vi "Save String Data to file.vi"(0 "Path":path, 5 "String to save":string, 7 "Header":string, 9 "Additional String":string, 12 "Disconnecting":bool) -> ()   [LabVIEW 2011]
panel:
  # "This vi saves data to file in a standard format\nData comes in as a 1D string\nA header is optional\nAn additional string can be added at the end of each line.\nThe path is the location of the data file.\n\n\nThe file is kept open at all times. When the software is to stop,\nthe disconnect is used to close the file properly.\nEvery 30 seconds, the file is flushed to empty the file buffer and\nforce the data to be actually saved to file - this is done to \nensure that only the last 30sec of data is lost if there is a power.\n\nThe file path is validated, the directory created if necessary and\nthe previous file closed if a new path file is specified."
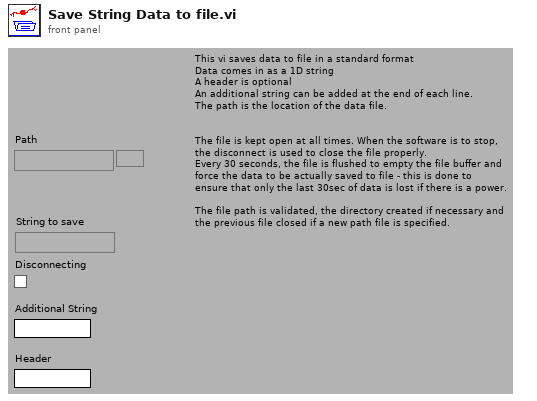
[diagram p1: front panel]
types:
  T1 = enum16{"open", "replace", "create", "open or create", "replace or create", "replace or create with confirmation"}
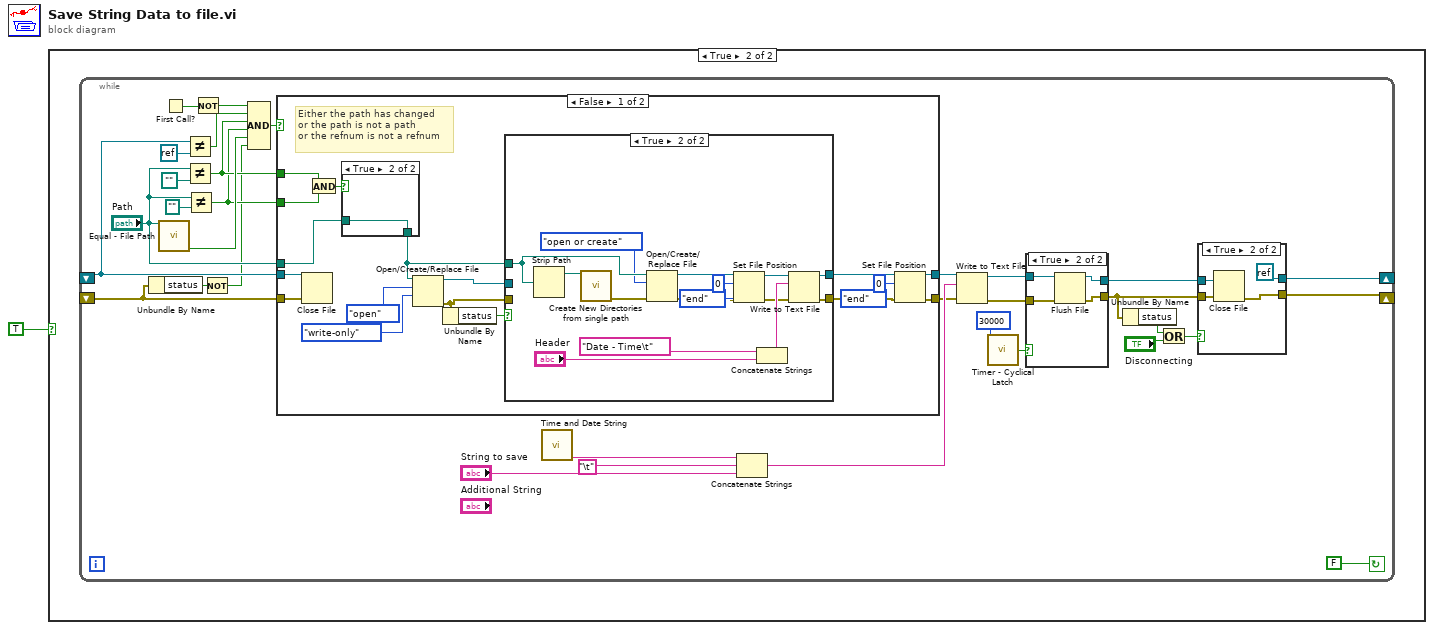
[diagram p0: block diagram]
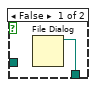
[diagram p5: hidden frame]
diagram:
  n1 = case shown="True" TRUE {
    frame False {
    }
    frame True {
      n2 = while {
        shift-left: _ -> [w11]
        shift-right: [w4] -> _
        shift-left: _ -> [w26]
        shift-right: [w28] -> _
        stop <- FALSE continue-if-true
        n3 = Unbundle By Name(w11) -> ("status"=w10:bool)
        n4 = call "Equal - File Path.vi"("Value In"="Path") -> ("Equal to previous value"=w21:bool)  [unwired: 13 in, 1 out]
        n5 = First Call?() -> (First Call?: T/F=w13:bool)
        n6 = Not Equal?(x=w26, y=refnum<k0> refnum) -> (x != y?=w25:bool)
        n7 = Not Equal?(x="Path", y=path "") -> (x != y?=w20:bool)
        n8 = Not Equal?(x="Path", y=path "") -> (x != y?=w19:bool)
        n9 = Not(x=w13) -> (.not. x?=w12:bool)
        n10 = Not(x=w10) -> (.not. x?=w9:bool)
        n11 = Compound Arithmetic op=AND(w12, w25, w20, w19, w21, w9) -> (w24:bool)
        n12 = case shown="False" w24 {
          tunnel: "Path" -> [w62 _]
          tunnel: [w49 w84] -> w2
          tunnel: [w52 w85] -> w3
          tunnel: w26 -> [w64 w85]
          tunnel: w11 -> [w63 w84]
          tunnel: w20 -> [w59 _]
          tunnel: w19 -> [w58 _]
          frame False {
            # "Either the path has changed\nor the path is not a path\nor the refnum is not a refnum"
            n13 = Close File(refnum=w64, error in=w63) -> ()  [unwired: 2 out]
            n14 = And(x=w59, y=w58) -> (x .and. y?=w60:bool)
            n15 = case shown="True" w60 {
              tunnel: w62 -> [_ w66]
              tunnel: [w65 w66] -> w61
              frame False {
                n16 = File Dialog() -> (3:w65:path)  [unwired: 7 in, 3 out]
              }
              frame True {
              }
            }
            n17 = Open/Create/Replace File(file path (use dialog)=w61, operation (0:open)=T1."open", access (0:read/write)=enum16{"read/write", "read-only", "write-only"}."write-only") -> (refnum out=w54:refnum<file>, error out=w53:errorcluster)  [unwired: 3 in, 1 out]
            n18 = Unbundle By Name(w53) -> ("status"=w57:bool)
            n19 = case shown="True" w57 {
              tunnel: w61 -> [_ w82]
              tunnel: w53 -> [w67 _]
              tunnel: w54 -> [w68 _]
              tunnel: [w68 w80] -> w51
              tunnel: [w67 w79] -> w50
              frame False {
              }
              frame True {
                n20 = Strip Path(path=w82) -> (stripped path=w83:path)  [unwired: 1 out]
                n21 = call "Create New Directories from single path.vi"("Create Directory Path"=w83) -> ("error out"=w81:errorcluster)  [unwired: 14 in]
                n22 = Open/Create/Replace File(file path (use dialog)=w82, error in=w81, operation (0:open)=T1."open or create") -> (refnum out=w73:refnum<file>, error out=w72:errorcluster)  [unwired: 3 in, 1 out]
                n23 = Set File Position(offset (in bytes) (0)=i64 0, refnum=w73, from (0:start)=enum16{"start", "end", "current"}."end", error in=w72) -> (refnum out=w70:refnum<file>, error out=w71:errorcluster)
                n24 = Concatenate Strings("Date - Time\t", "Header") -> (w77:string)
                n25 = Write to Text File(file (use dialog)=w70, text=w77, error in=w71) -> (refnum out=w80:refnum<file>, error out=w79:errorcluster)  [unwired: 1 in, 1 out]
              }
            }
            n26 = Set File Position(offset (in bytes) (0)=i64 0, refnum=w51, from (0:start)=enum16{"start", "end", "current"}."end", error in=w50) -> (refnum out=w52:refnum<file>, error out=w49:errorcluster)
          }
          frame True {
            # "Path is real\nPath is the same as the previous path\nFile refnum is not equal to \"Not a refnum\""
          }
        }
        n27 = call "Time and Date String.vi"() -> ("date and time string"=w18:string)  [unwired: 13 in, 2 out]
        n28 = Concatenate Strings(w18, "\t", "String to save") -> (w16:string)
        n29 = Write to Text File(file (use dialog)=w3, text=w16, error in=w2) -> (refnum out=w33:refnum<file>, error out=w32:errorcluster)  [unwired: 1 in, 1 out]
        n30 = call "Timer - Cyclical Latch.vi"("Timer (msec)"=u32 30000) -> ("Timer Trigger"=w30:bool)  [unwired: 14 in]
        n31 = case shown="True" w30 {
          tunnel: w33 -> [w42 w46]
          tunnel: w32 -> [w41 w45]
          tunnel: [w42 w44] -> w31
          tunnel: [w41 w43] -> w8
          frame False {
          }
          frame True {
            n32 = Flush File(refnum=w46, error in=w45) -> (refnum out=w44:refnum<file>, error out=w43:errorcluster)
          }
        }
        n33 = Unbundle By Name(w8) -> ("status"=w6:bool)
        n34 = Or(x=w6, y="Disconnecting") -> (x .or. y?=w7:bool)
        n35 = case shown="True" w7 {
          tunnel: w31 -> [w35 w40]
          tunnel: w8 -> [w36 w39]
          tunnel: [w36 w38] -> w4
          tunnel: [w35 refnum<k0> refnum] -> w28
          frame False {
          }
          frame True {
            n36 = Close File(refnum=w40, error in=w39) -> (error out=w38:errorcluster)  [unwired: 1 out]
          }
        }
      }
    }
  }
